vi "应用举例（映射表）.vi"() -> ()   [LabVIEW 2012]
panel:
  in  "映射表":u8[](array[numeric])=[149, 131, 111, 218, 161, 223, 167, 96, 220, 194, 178, 70, 162, 32, 128, 158, 14, 135, 242, 151, 35, 236, 79, 213, 168, 202, 105, 69, 143, 172, 51, 73, 67, 20, 248, 235, 48, 41, 212, 85, 241, 90, 123, 91, 110, 29, 118, 254, 68, 246, 100, 87, 219, 157, 7, 17, 66, 94, 120, 55, 75, 240, 145, 109, 54, 141, 82, 1, 127, 146, 3, 22, 193, 81, 227, 65, 150, 6, 132, 189, 229, 83, 214, 148, 12, 226, 113, 25, 74, 176, 58, 101, 185, 27, 98, 50, 197, 204, 224, 233, 152, 228, 63, 243, 18, 4, 190, 57, 155, 53, 62, 163, 23, 122, 124, 217, 46, 255, 16, 187, 112, 102, 169, 133, 200, 59, 191, 13, 31, 33, 139, 231, 92, 137, 232, 103, 210, 24, 177, 249, 78, 142, 159, 134, 247, 116, 199, 165, 34, 245, 222, 47, 144, 56, 130, 195, 196, 170, 225, 38, 198, 126, 15, 10, 76, 2, 108, 11, 121, 64, 239, 203, 21, 154, 37, 39, 117, 206, 140, 138, 174, 188, 72, 180, 156, 173, 99, 252, 5, 129, 36, 147, 221, 251, 80, 211, 19, 215, 237, 77, 183, 208, 9, 238, 43, 253, 42, 52, 28, 45, 104, 8, 160, 184, 95, 61, 97, 40, 106, 44, 71, 93, 153, 205, 164, 201, 30, 86, 136, 26, 244, 179, 171, 175, 107, 250, 234, 186, 119, 216, 192, 0, 166, 182, 230, 49, 60, 207, 125, 114, 88, 209, 89, 84, 181, 115]
  out "加密后字符串":string
  in  "输入字符串":string
  out "解密字符串":string
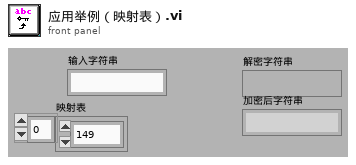
[diagram p1: front panel]
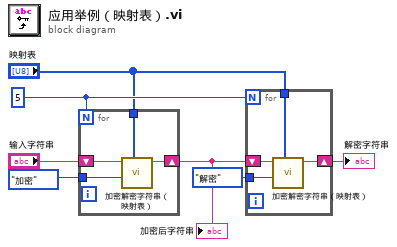
[diagram p0: block diagram]
diagram:
  w4 = 5
  n1 = for {
    N: w4 -> [_]
    tunnel: enum16{"加密", "解密"}."加密" ("模式") -> [w10]
    shift-right: [w9] -> w5
    shift-left: "输入字符串" -> [w11]
    tunnel: "映射表" -> [w8]
    n2 = call "加密解密字符串（映射表）.vi"("映射表"=w8, "模式"=w10, "输入字符串"=w11) -> ("输出字符串"=w9:string)  [unwired: 7 in, 1 out]
  }
  "加密后字符串" <- w5
  n3 = for {
    N: w4 -> [_]
    tunnel: enum16{"加密", "解密"}."解密" ("模式") -> [w15]
    shift-right: [w13] -> w3
    shift-left: w5 -> [w14]
    tunnel: "映射表" -> [w12]
    n4 = call "加密解密字符串（映射表）.vi"("映射表"=w12, "模式"=w15, "输入字符串"=w14) -> ("输出字符串"=w13:string)  [unwired: 7 in, 1 out]
  }
  "解密字符串" <- w3
